vi "Transfer Required Buffer Size.vi"(8 "error in (no error)":errorcluster, 11 "Transfer Configuration in":T1 {"channel configurations"."buffer offset" format="%d bytes"}) -> (0 "error out":errorcluster, 2 "required buffer size":u64 format="%d bytes", 3 "Transfer Configuration out":T1 {"channel configurations"."buffer offset" format="%d bytes"})   [LabVIEW 2017, in "DSF Core.lvlib"]
uses:
  DSF Core.lvlib
  Controls/DSF Engine Transfer Configuration.ctl
  Controls/DSF Byte Order.ctl
  Controls/DSF Engine Channel Configuration.ctl
  Controls/DSF Data Type.ctl
  Controls/DSF Settings Info.ctl
  Shared/VIs/Sizeof.vi
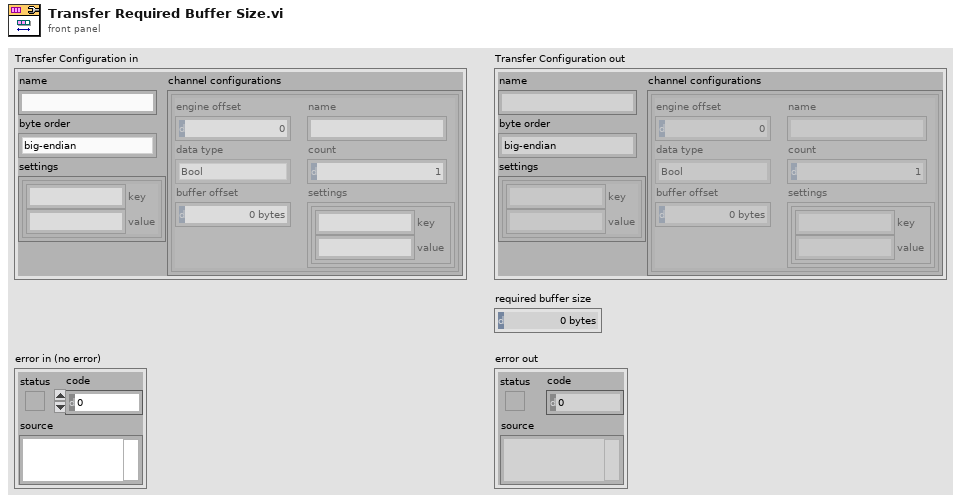
[diagram p1: front panel]
types:
  T1 = typedef "DSF Core.lvlib/DSF Engine Transfer Configuration.ctl" = cluster{"name":string, "byte order":T2, "channel configurations":T3[], "settings":T5}
  T2 = typedef "DSF Core.lvlib/DSF Byte Order.ctl" = enum8{"big-endian", "little-endian"}
  T3 = typedef "DSF Core.lvlib/DSF Engine Channel Configuration.ctl" = cluster{"engine offset":u64, "name":string, "data type":T4, "count":u64, "buffer offset":u64, "settings":T5}
  T4 = typedef "DSF Core.lvlib/DSF Data Type.ctl" = enum8{"Bool", "SGL", "DBL", "I8", "I16", "I32", "I64", "U8", "U16", "U32", "U64"}
  T5 = typedef "DSF Core.lvlib/DSF Settings Info.ctl" = cluster{"key":string, "value":string}[]
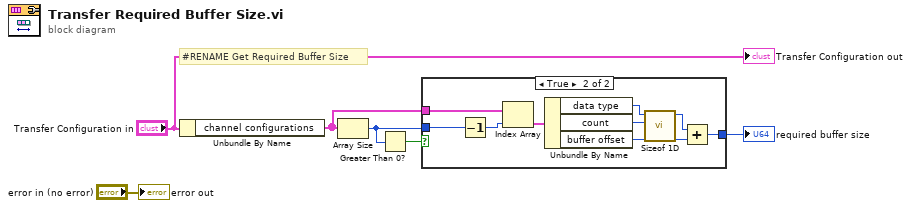
[diagram p0: block diagram]
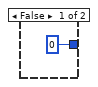
[diagram p2: hidden frame]
diagram:
  # "#RENAME Get Required Buffer Size"
  n1 = Unbundle By Name("Transfer Configuration in") -> ("channel configurations"=w1:T3[])
  n2 = Array Size(array=w1) -> (size(s)=w5:i32)
  n3 = Greater Than 0?(x=w5) -> (x > 0?=w4:bool)
  n4 = case shown="True" w4 {
    tunnel: w5 -> [_ w16]
    tunnel: w1 -> [_ w15]
    tunnel: [u64 0 w8] -> w3
    frame False {
    }
    frame True {
      n5 = Decrement(x=w16) -> (x-1=w14:i32)
      n6 = Index Array(array=w15, index=w14) -> (element=w13:T3)
      n7 = Unbundle By Name(w13) -> ("data type"=w12:T4, "count"=w11:u64, "buffer offset"=w10:u64)
      n8 = call "Sizeof 1D.vi"("count"=w11, "data type"=w12) -> ("size in bytes"=w9:u64)  [unwired: 9 in]
      n9 = Add(x=w9, y=w10) -> (x+y=w8:u64)
    }
  }
  "required buffer size" <- w3
  "error out" <- "error in (no error)"
  "Transfer Configuration out" <- "Transfer Configuration in"
